vi "Save changes.vi"(6 "Defer restart? (true)":bool=TRUE, 8 "error in (no error)":errorcluster, 11 "RT Management in":refnum<class "RT Management.lvclass">) -> (0 "error out":errorcluster, 3 "RT Management out":refnum<class "RT Management.lvclass">)   [LabVIEW 2016, in "RT Management.lvlib" / "RT Management.lvclass"]
doc: "Saves any changes set on the target session. Some changes require restarts. In those cases, the user can specifiy to defer the needed restart, which can then be called manually or will be ran automatically when the Close method is called if a needed restart has not occurred."
uses:
  RT Management.lvclass
  RT Management.lvclass/RT Management.ctl
  Get SysCfg Session.vi
  Set Restart needed.vi
  <vilib>/nisyscfg/Save Changes (Hardware).vi
  <vilib>/nisyscfg/Close (Hardware).vi
  <vilib>/nisyscfg/Save Changes (System).vi
  <vilib>/nisyscfg/nisyscfg.lvlib
  <resource>/objmgr/nisysapi.rc
  <resource>/objmgr/nicriosae.rc
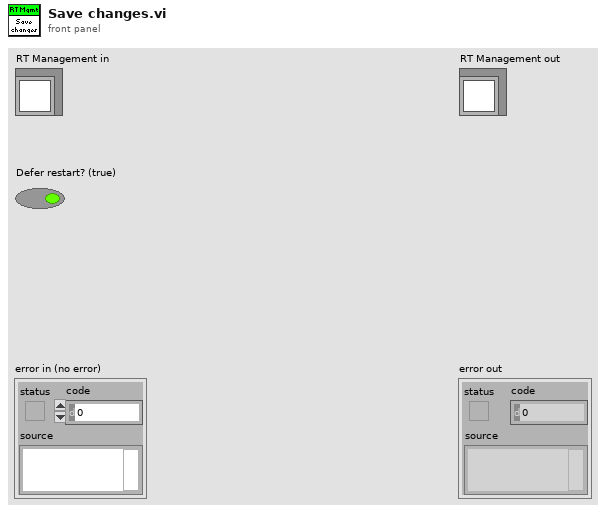
[diagram p1: front panel]
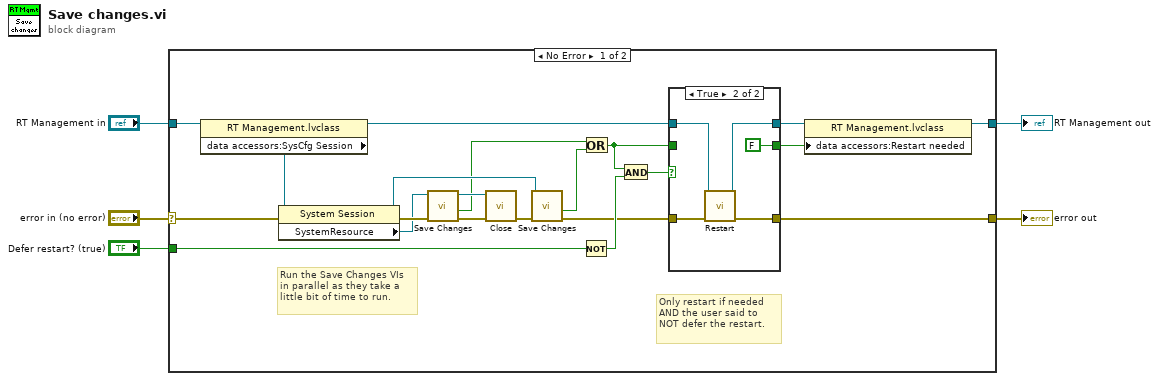
[diagram p0: block diagram]
diagram:
  n1 = case shown="No Error" "error in (no error)" {
    selector: "error in (no error)" -> [w26 w36]
    tunnel: [w24 w36] -> w4
    tunnel: [w22 w35] -> w2
    tunnel: "RT Management in" -> [w23 w35]
    tunnel: "Defer restart? (true)" -> [w21 _]
    frame No Error {
      # "Run the Save Changes VIs in parallel as they take a little bit of time to run."
      # "Only restart if needed AND the user said to NOT defer the restart."
      n2 = property class="RT Management.lvclass"(reference=w23) -> (reference out=w20:refnum<class "RT Management.lvclass">, "data accessors:SysCfg Session"=w8:refnum<k21>)  [unwired: 1 in, 1 out]
      n3 = property class="System Session"(reference=w8, error in=w26) -> (reference out=w7:refnum<k21>, error out=w12:errorcluster, "SystemResource"=w9:refnum<k20>)
      n4 = call-poly <vilib>:"Save Changes.vi"("error in (no error)"=w12, "Resource in"=w9) -> ("error out"=w11:errorcluster, "Changes Require Restart"=w6:bool, "Resource out"=w10:refnum<k20>)  [unwired: 6 in, 1 out]
      n5 = call-poly <vilib>:"Close.vi"("error in (no error)"=w11, "Resource in"=w10) -> ("error out"=w15:errorcluster)  [unwired: 9 in]
      n6 = call-poly <vilib>:"Save Changes.vi"("error in (no error)"=w15, "Session in"=w7) -> ("error out"=w14:errorcluster, "Changes Require Restart"=w13:bool)  [unwired: 6 in, 2 out]
      n7 = Not(x=w21) -> (.not. x?=w16:bool)
      n8 = Or(x=w6, y=w13) -> (x .or. y?=w17:bool)
      n9 = And(x=w17, y=w16) -> (x .and. y?=w25:bool)
      n10 = case shown="True" w25 {
        tunnel: w14 -> [w29 w34]
        tunnel: [w29 w33] -> w24
        tunnel: w20 -> [w28 w32]
        tunnel: [w28 w31] -> w19
        tunnel: [w27 FALSE] -> w18
        tunnel: w17 -> [w27 _]
        frame False {
        }
        frame True {
          n11 = call "Restart.vi"("error in (no error)"=w34, "RT Management in"=w32) -> ("error out"=w33:errorcluster, "RT Management out"=w31:refnum<class "RT Management.lvclass">)  [unwired: 7 in]
        }
      }
      n12 = property class="RT Management.lvclass"(reference=w19, "data accessors:Restart needed"=w18) -> (reference out=w22:refnum<class "RT Management.lvclass">)  [unwired: 1 in, 1 out]
    }
    frame Error {
    }
  }
  "error out" <- w4
  "RT Management out" <- w2
